vi "Feature Vector State Action.vi"(8 "n x(s, a)":i32=3, 10 "action":dbl, 11 "state":dbl[](array[numeric])=[0.46211715726000974, 0.46211715726000974, 0.7071067811865475]) -> (3 "x(s, a)":dbl[](array[numeric])=[1.0, -0.6056998670788134, -0.26625534204141565, 0.11873171128012475, -0.8619805458075959, 0.9254712927602428, -0.9718055614729862, 0.40101101649098936, 0.4860209227015219, 0.11873171128012475, -0.8619805458075959, 0.9254712927602428, -0.9718055614729862, 0.40101101649098936, 0.4860209227015219, -0.3494999859705848, 0.9572059942679109, -0.8100591010196486, -0.9718055614729862, 0.40101101649098936, 0.4860209227015219, -0.3494999859705848, 0.9572059942679109, -0.8100591010196486, 0.8888120986196519, -0.17370960499694593, -0.678380329305727])   [LabVIEW 2017]
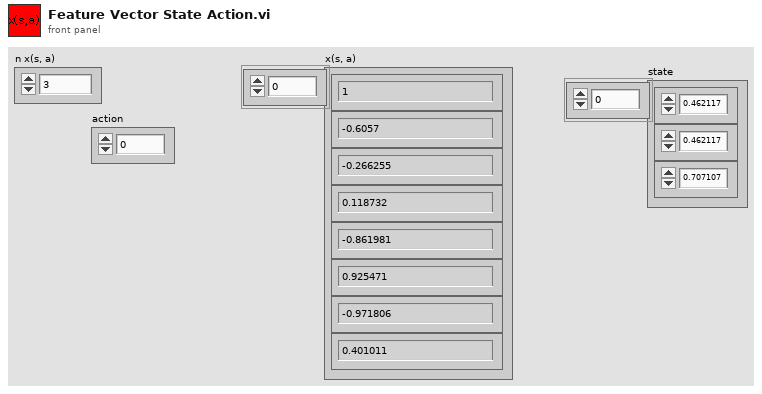
[diagram p1: front panel]
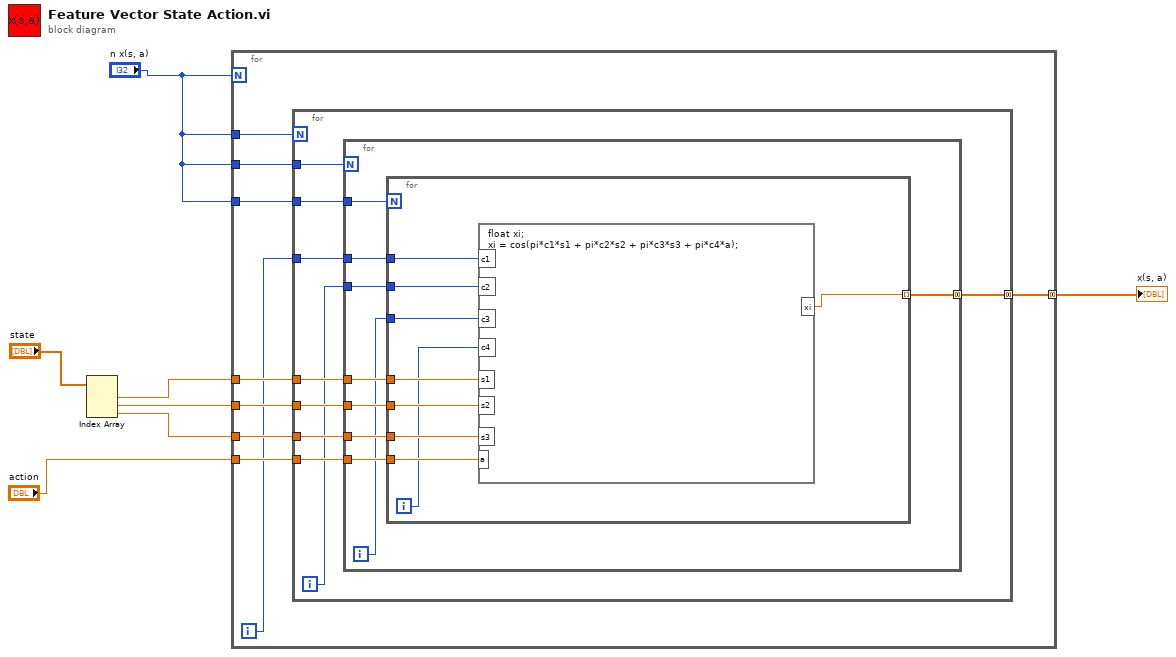
[diagram p0: block diagram]
diagram:
  n1 = Index Array(array="state") -> (element #1=w5:dbl, element #2=w4:dbl, element #3=w3:dbl)  [unwired: 3 in]
  n2 = for {
    N: "n x(s, a)" -> [_]
    tunnel: "n x(s, a)" -> [w16]
    tunnel: "n x(s, a)" -> [w15]
    tunnel: "n x(s, a)" -> [w14]
    tunnel: w5 -> [w13]
    tunnel: w4 -> [w12]
    tunnel: w3 -> [w11]
    tunnel: "action" -> [w10]
    tunnel: [w8] -> w1 mode=concatenating
    i -> [w9]
    n3 = for {
      N: w16 -> [_]
      tunnel: w15 -> [w25]
      tunnel: w14 -> [w24]
      tunnel: w13 -> [w23]
      tunnel: w12 -> [w22]
      tunnel: w11 -> [w21]
      tunnel: w10 -> [w20]
      tunnel: w9 -> [w19]
      tunnel: [w17] -> w8 mode=concatenating
      i -> [w18]
      n4 = for {
        N: w25 -> [_]
        tunnel: w24 -> [w34]
        tunnel: w23 -> [w33]
        tunnel: w22 -> [w32]
        tunnel: w21 -> [w31]
        tunnel: w20 -> [w30]
        tunnel: w19 -> [w29]
        tunnel: w18 -> [w28]
        tunnel: [w26] -> w17 mode=concatenating
        i -> [w27]
        n5 = for {
          N: w34 -> [_]
          tunnel: w33 -> [w43]
          tunnel: w32 -> [w42]
          tunnel: w31 -> [w41]
          tunnel: w30 -> [w40]
          tunnel: w29 -> [w39]
          tunnel: w28 -> [w38]
          tunnel: w27 -> [w37]
          tunnel: [w35] -> w26 mode=indexing
          i -> [w36]
          n6 = formula code="float xi;\nxi = cos(pi*c1*s1 + pi*c2*s2 + pi*c3*s3 + pi*c4*a);"("c1"=w39, "c2"=w38, "c3"=w37, "s1"=w43, "s2"=w42, "s3"=w41, "c4"=w36, "a"=w40) -> ("xi"=w35:dbl)
        }
      }
    }
  }
  "x(s, a)" <- w1
